vi "Read AI Single Command2Data.vi"(11 "Teszt cluster":T1) -> (1 "Min":dbl, 2 "Max":dbl, 3 "Channel Name":string)   [LabVIEW 2014]
uses:
  Teszt/Teszt.ctl
  Teszt/Command.ctl
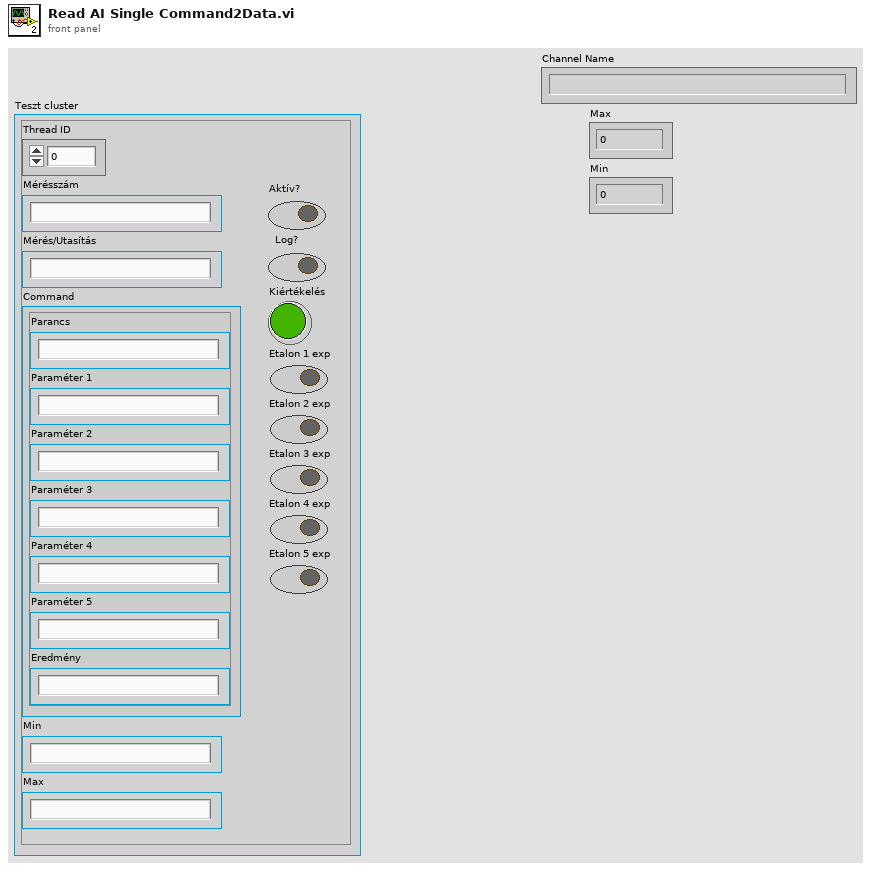
[diagram p1: front panel]
types:
  T1 = typedef "Teszt.ctl" = cluster{"Thread ID":dbl, "Mérésszám":string, "Mérés/Utasítás":string, "Command":T2, "Min":string, "Max":string, "Aktív?":bool, "Log?":bool, "Kiértékelés":bool, "Etalon 1 exp":bool, "Etalon 2 exp":bool, "Etalon 3 exp":bool, "Etalon 4 exp":bool, "Etalon 5 exp":bool}
  T2 = typedef "Command.ctl" = cluster{"Parancs":string, "Paraméter 1":string, "Paraméter 2":string, "Paraméter 3":string, "Paraméter 4":string, "Paraméter 5":string, "Eredmény":string}
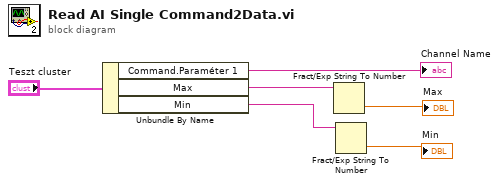
[diagram p0: block diagram]
diagram:
  n1 = Unbundle By Name("Teszt cluster") -> ("Command.Paraméter 1"=→"Channel Name":string, "Max"=w5:string, "Min"=w4:string)
  n2 = Fract/Exp String To Number(string=w5) -> (number=→"Max":dbl)  [unwired: 3 in, 1 out]
  n3 = Fract/Exp String To Number(string=w4) -> (number=→"Min":dbl)  [unwired: 3 in, 1 out]
